vi "测试-生成word报表.vi"() -> ()   [LabVIEW 2018]
uses:
  <vilib>/Utility/NIReport.llb/Report Type.ctl
  <vilib>/Utility/NIReport.llb/Append Report Text (str wrap).vi
  <vilib>/Utility/NIReport.llb/NI_report.lvclass
  <vilib>/Utility/NIReport.llb/NI_ReportGenerationCore.lvlib
panel:
  in  "合格性":string="合格"
  in  "检验人":string
  in  "类型":string="类型1"
  in  "部位":string="位置1"
  in  "输入产品序号":string
  out "保存路径":path
  out "检查文件路径是否正确":bool caption="文件或文件夹存在？"
  out "模板路径":path
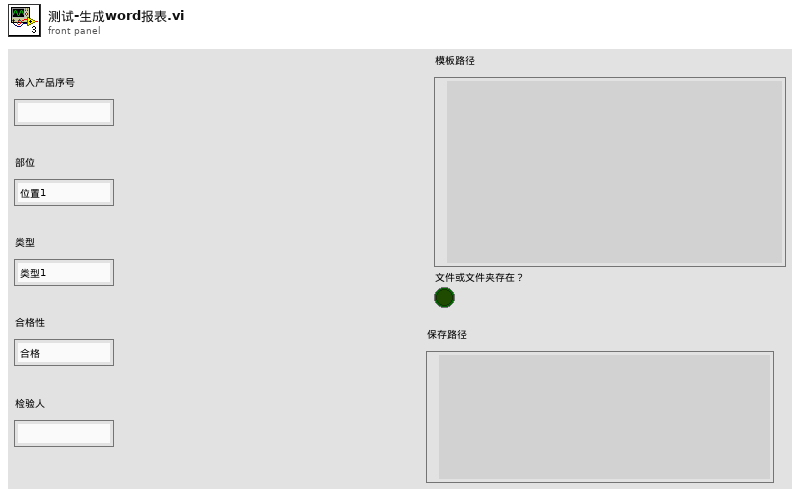
[diagram p1: front panel]
types:
  T1 = typedef "NI_ReportGenerationCore.lvlib/Report Type.ctl" = enum16{"HTML", "Word", "Excel"}
  T2 = cluster{"position (excel)":cluster{"row":i32, "column":i32}, "name (excel)":string, "bookmark (word)":string}
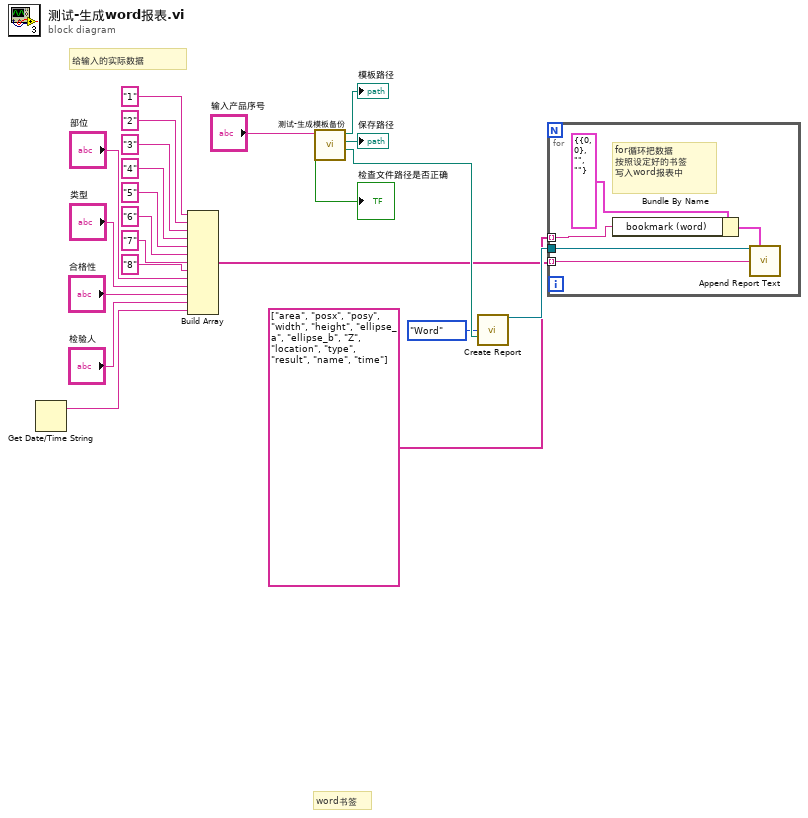
[diagram p0: block diagram]
diagram:
  # "word书签"
  # "给输入的实际数据"
  n1 = Get Date/Time String() -> (date string=w4:string)  [unwired: 3 in, 1 out]
  n2 = Build Array("1", "2", "3", "4", "5" ("元素"), "6" ("元素"), "7" ("元素"), "8" ("元素"), "部位", "类型", "合格性", "检验人", w4) -> (w15:string[])
  n3 = call "测试-生成模板备份.vi"("输入产品序号"="输入产品序号") -> ("new path"=w21:path, "保存路径"=→"保存路径":path, "模板路径"=→"模板路径":path, "检查文件路径是否正确"=→"检查文件路径是否正确":bool)  [unwired: 7 in]
  n4 = call <vilib>:"Create Report.vi"("report type"=Report_Type."Word", "template (empty)"=w21) -> ("report out"=w22:refnum<class "NI_report.lvclass">)  [unwired: 12 in, 1 out]
  n5 = for {
    tunnel: w22 -> [w27]
    tunnel: string[] ["area", "posx", "posy", "width", "height", "ellipse_a", "ellipse_b", "Z", "location", "type", "result", "name", "time"] -> [w25] mode=indexing
    tunnel: w15 -> [w23] mode=indexing
    # "for循环把数据\n按照设定好的书签 \n写入word报表中"
    n6 = Bundle By Name(cluster=T2 {"position (excel)"={"row"=0, "column"=0}, "name (excel)"="", "bookmark (word)"=""} ("MS Office parameters"), "bookmark (word)"=w25) -> (w24:T2)
    n7 = call-poly <vilib>:"Append Report Text.vi"("report in"=w27, "MS Office parameters"=w24, "text"=w23) -> ()  [unwired: 9 in, 4 out]
  }
